vi "Initialize.vi"(0 "VISA resource name":refnum<visa-resource-name>, 1 "ID Query (True)":bool=TRUE, 2 "Reset (False)":bool, 3 "error in (no error)":errorcluster, 4 "Serial Link (RS232)":enum16{"RS232", "USB"}(ring)) -> (7 "VISA resource name out":refnum<visa-resource-name>, 10 "error out":errorcluster {"code" format="%.0x"})   [LabVIEW 2019, in "Newport ESP301.lvlib"]
doc: "Establishes communication with the instrument and optionally performs an instrument identification query and/or an instrument reset. It also places the instrument in a default state needed for other instrument driver operations. Therefore, call this VI before calling other instrument driver VIs for this instrument. Generally, you need to call the Initialize VI only once at the beginning of an application."
uses:
  Newport ESP301.lvlib
panel:
  # "(c) 2009 - 2013 Newport Corporation"
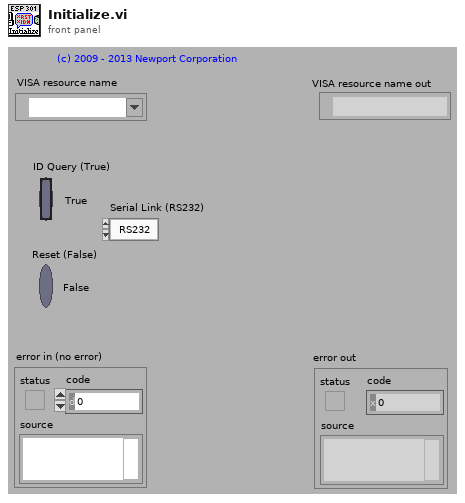
[diagram p1: front panel]
types:
  T1 = cluster{"Baud Rate":u32, "Parity":u16, "Data Bits":u16, "Stop Bits":u16, "Flow Control":u16}
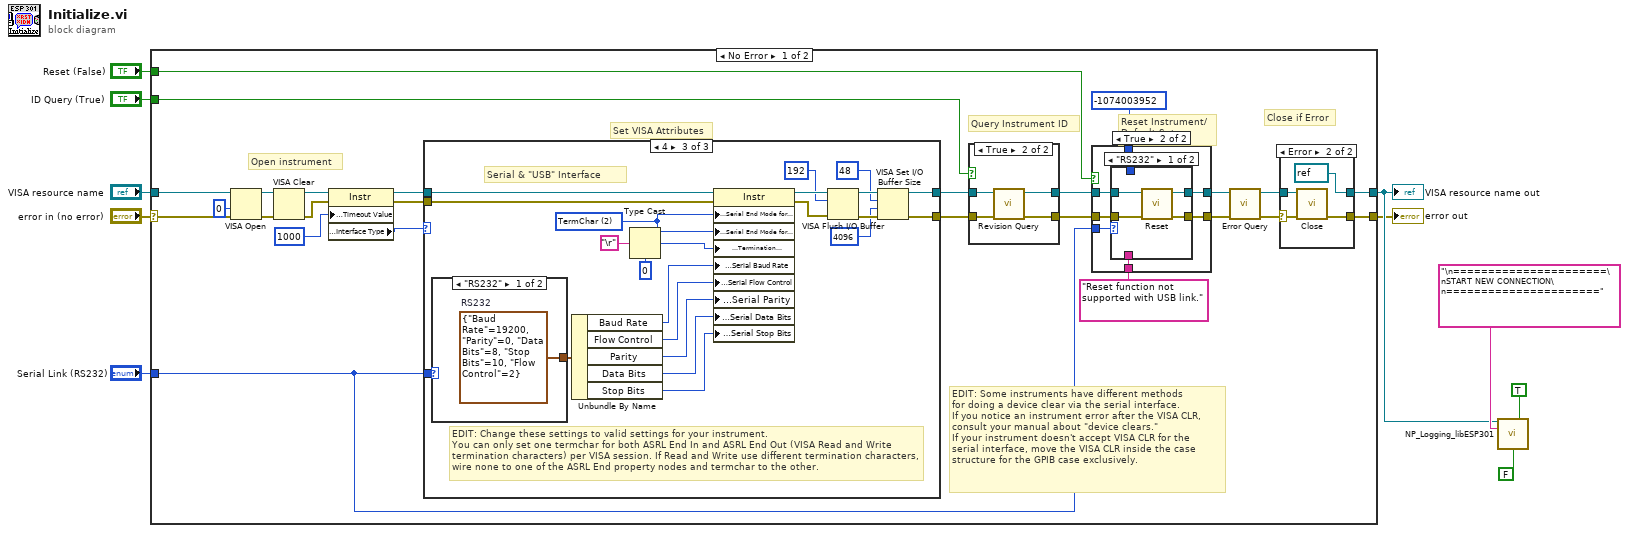
[diagram p0: block diagram]
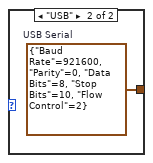
[diagram p5: hidden frame]
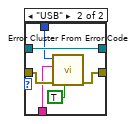
[diagram p7: hidden frame]
diagram:
  n1 = case shown="No Error" "error in (no error)" {
    selector: "error in (no error)" -> [w18 w97]
    tunnel: "ID Query (True)" -> [w34 _]
    tunnel: "Reset (False)" -> [w33 _]
    tunnel: "VISA resource name" -> [w32 w96]
    tunnel: [w14 w96] -> w2
    tunnel: [w16 w97] -> w1
    tunnel: "Serial Link (RS232)" -> [w13 _]
    frame No Error {
      # "EDIT: Some instruments have different methods\nfor doing a device clear via the serial interface.  \nIf you notice an instrument error after the VISA CLR,\nconsult your manual about \"device clears.\"  \nIf your instrument doesn't accept VISA CLR for the\nserial interface, move the VISA CLR inside the case \nstructure for the GPIB case exclusively."
      # "Set VISA Attributes"
      # "Close if Error"
      # "Query Instrument ID"
      # "Reset Instrument/\nDefault Setup"
      # "Open instrument"
      n2 = VISA Open(access mode=u32 0, error in (no error)=w18, VISA resource name=w32) -> (VISA resource name=w25:refnum<visa-resource-name>, error out=w24:errorcluster)  [unwired: 2 out]
      n3 = VISA Clear(VISA resource name=w25, error in (no error)=w24) -> (VISA resource name out=w23:refnum<visa-resource-name>, error out=w22:errorcluster)
      n4 = property class="Instr"(reference=w23, error in=w22, "General Settings:Timeout Value"=u32 1000) -> (reference out=w28:refnum<visa-resource-name>, error out=w27:errorcluster, "Interface Information:Interface Type"=w19:u16)
      n5 = case shown="4" w19 {
        tunnel: [w43 w46 w65] -> w30
        tunnel: [w44 w45 w62] -> w29
        tunnel: w28 -> [w43 w46 w67]
        tunnel: w27 -> [w44 w45 w68]
        tunnel: w13 -> [_ _ w49]
        frame Default {
          # "TCP/IP, and USB Interface"
        }
        frame 1 {
          # "GPIB Interface"
        }
        frame 4 {
          w56 = u16 2 items=["None", "LastBit", "TermChar"] ("Serial Settings:Serial End Mode for Reads")
          # "EDIT: Change these settings to valid settings for your instrument.\nYou can only set one termchar for both ASRL End In and ASRL End Out (VISA Read and Write termination characters) per VISA session. If Read and Write use different termination characters, wire none to one of the ASRL End property nodes and termchar to the other."
          # "Serial & \"USB\" Interface"
          n6 = case shown="\"RS232\"" w49 {
            tunnel: [w69 w70] -> w48
            frame "RS232" {
              w69 = T1 {"Baud Rate"=19200, "Parity"=0, "Data Bits"=8, "Stop Bits"=10, "Flow Control"=2}  # RS232
            }
            frame "USB" {
              w70 = T1 {"Baud Rate"=921600, "Parity"=0, "Data Bits"=8, "Stop Bits"=10, "Flow Control"=2}  # USB Serial
            }
          }
          n7 = Unbundle By Name(w48) -> ("Baud Rate"=w54:u32, "Flow Control"=w51:u16, "Parity"=w52:u16, "Data Bits"=w53:u16, "Stop Bits"=w50:u16)
          n8 = Type Cast(type=u8 0, x="\r") -> (*(type *) &x=w55:u8)
          n9 = property class="Instr"(reference=w67, error in=w68, "Serial Settings:Serial End Mode for Reads"=w56, "Serial Settings:Serial End Mode for Writes"=w56, "Message Based Settings:Termination Character"=w55, "Serial Settings:Serial Baud Rate"=w54, "Serial Settings:Serial Flow Control"=w51, "Serial Settings:Serial Parity"=w52, "Serial Settings:Serial Data Bits"=w53, "Serial Settings:Serial Stop Bits"=w50) -> (reference out=w61:refnum<visa-resource-name>, error out=w64:errorcluster)
          n10 = VISA Flush I/O Buffer(VISA resource name=w61, mask (16)=u16 192, error in (no error)=w64) -> (VISA resource name out=w66:refnum<visa-resource-name>, error out=w63:errorcluster)
          n11 = VISA Set I/O Buffer Size(VISA resource name=w66, mask (16)=u16 48, size (4096)=u32 4096 ("size (0)"), error in (no error)=w63) -> (VISA resource name out=w65:refnum<visa-resource-name>, error out=w62:errorcluster)
        }
      }
      n12 = case shown="True" w34 {
        tunnel: [w90 w92] -> w35
        tunnel: [w91 w94] -> w36
        tunnel: w30 -> [w91 w95]
        tunnel: w29 -> [w90 w93]
        frame False {
        }
        frame True {
          n13 = call "Revision Query.vi"("error in (no error)"=w93, "VISA resource name"=w95) -> ("error out"=w92:errorcluster, "VISA resource name out"=w94:refnum<visa-resource-name>)  [unwired: 8 out]
        }
      }
      n14 = case shown="True" w33 {
        tunnel: w35 -> [w71 w76]
        tunnel: [w71 w79] -> w20
        tunnel: w36 -> [w72 w77]
        tunnel: [w72 w78] -> w21
        tunnel: w13 -> [_ w75]
        tunnel: -1074003952 ("Code") -> [_ w74]
        tunnel: "Reset function not supported with USB link." ("Source (VI Name)") -> [_ w73]
        frame False {
        }
        frame True {
          n15 = case shown="\"RS232\"" w75 {
            tunnel: [w83 w86] -> w79
            tunnel: [w82 w89] -> w78
            tunnel: w77 -> [w81 w89]
            tunnel: w76 -> [w80 w87]
            tunnel: w74 -> [_ w85]
            tunnel: w73 -> [_ w84]
            frame "RS232" {
              n16 = call "Reset.vi"("error in (no error)"=w80, "VISA resource name"=w81) -> ("error out"=w83:errorcluster, "VISA resource name out"=w82:refnum<visa-resource-name>)  [unwired: 4 out]
            }
            frame "USB" {
              n17 = call <vilib>:"Error Cluster From Error Code.vi"("show call chain? (False)"=TRUE, "error in (no error)"=w87, "error message (\"\")"=w84, "error code (0)"=w85) -> ("error out"=w86:errorcluster)  [unwired: 5 out]
            }
          }
        }
      }
      n18 = call "Error Query.vi"("error in (no error)"=w20, "VISA resource name"=w21) -> ("error out"=w17:errorcluster, "VISA resource name out"=w15:refnum<visa-resource-name>)  [unwired: 4 out]
      n19 = case shown="Error" w17 {
        selector: w17 -> [w38 w40]
        tunnel: w15 -> [w37 w41]
        tunnel: [w37 refnum<visa-resource-name> refnum ("VISA resource name out")] -> w14
        tunnel: [w38 w42] -> w16
        frame No Error {
        }
        frame Error {
          n20 = call "Close.vi"("error in (no error)"=w40, "VISA resource name"=w41) -> ("error out"=w42:errorcluster)  [unwired: 9 out]
        }
      }
    }
    frame Error {
    }
  }
  "VISA resource name out" <- w2
  "error out" <- w1
  n21 = call "NP_Logging_libESP301.vi"("Instrument Channel"=w2, "Generic Strings"=TRUE, "String 1 {Write} (in)"="\n======================\nSTART NEW CONNECTION\n======================", "String 2 Enable (T)"=FALSE) -> ()  [unwired: 8 in, 4 out]
